vi "transmitRFID_noASK.vi"() -> ()   [LabVIEW 2015]
uses:
  <instrlib>/niUSRP/niUSRP Write Tx Data (I16).vi
panel:
  out "Loop":i32
  in  "Symbol Rate [Hz]":dbl=10000000.0 format="%#_13p"
  in  "Parameters Select":T1={"Target"=7, "Action"=0, "MemBank"=1, "truncate"=FALSE} {"MemBank" items=["00 RFU", "01 EPC", "10 TID", "11 User"]; "Action" items=["000", "001", "010", "011", "100", "101", "110", "111"]; "Target" items=["000 Inventoried (S0)", "001 Inventoried (S1)", "010 Inventoried (S2)", "011 Inventoried (S3)", "100 SL", "101 RFU", "110 RFU", "111 RFU"]}
  in  "Parameters Symbols":T2={"Tari"=2.5e-05, "PW"=0.5, "factor for \"1\" symbol"=0.5, "RTcal"=2.5, "TRcal"=2.5, "Delimiter"=1.25e-05} {"TRcal" min=1.1 max=3.0 step=0.1; "RTcal" min=2.5 max=3.0 step=0.1; "factor for \"1\" symbol" min=0.5 max=1.0 step=0.1; "PW" min=0.265 max=0.525 step=0.001; "Tari" format="%#_3p"}
  out "coerced IQ rate":dbl=100000.0 format="%#_6p"
  out "carrier frequency":dbl=100000.0 format="%#_6p"
  out "coerced gain":dbl format="%#_6f"
  out "error out":errorcluster
  in  "stop":bool
  in  "IQ rate":dbl=100000.0 format="%#_6p"
  in  "carrier frequency":dbl=100000.0 format="%#_6p"
  in  "gain":dbl format="%#_6f"
  in  "tx device names":refnum<k15>
  # "Transmit RFID"
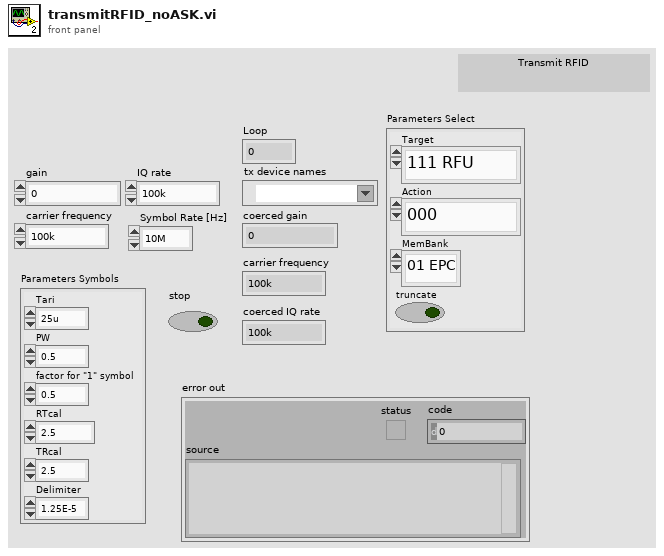
[diagram p1: front panel]
types:
  T1 = cluster{"Target":u16, "Action":u16, "MemBank":u16, "truncate":bool}
  T2 = cluster{"Tari":dbl, "PW":dbl, "factor for \"1\" symbol":dbl, "RTcal":dbl, "TRcal":dbl, "Delimiter":dbl}
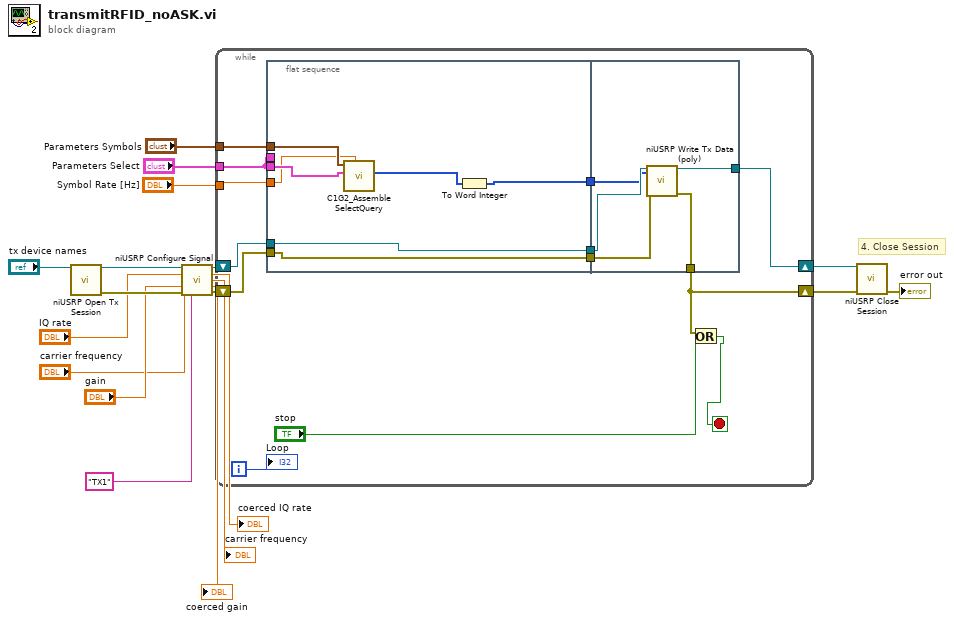
[diagram p0: block diagram]
diagram:
  # "4. Close Session"
  n1 = call <instrlib>:"niUSRP Open Tx Session.vi"("device names"="tx device names") -> ("session handle out"=w18:refnum<k15>, "error out"=w17:errorcluster)  [unwired: 13 in]
  n2 = call <instrlib>:"niUSRP Configure Signal.vi"("session handle"=w18, "IQ rate"="IQ rate", "carrier frequency"="carrier frequency", "gain"="gain", "error in (no error)"=w17, "active antenna"="TX1") -> ("session handle out"=w12:refnum<k15>, "coerced IQ rate"=→"coerced IQ rate":dbl, "coerced carrier frequency"=→"carrier frequency":dbl, "coerced gain"=→"coerced gain":dbl, "error out"=w11:errorcluster)  [unwired: 5 in]
  n3 = while {
    shift-right: [w26] -> w10
    shift-left: w12 -> [w23]
    shift-right: [w25] -> w9
    shift-left: w11 -> [w22]
    tunnel: "Parameters Symbols" -> [w27]
    tunnel: "Parameters Select" -> [w20]
    tunnel: "Symbol Rate [Hz]" -> [w28]
    i -> [w29]
    stop <- w31 stop-if-true
    n4 = flat-sequence {
      tunnel: w28 -> [w32]
      tunnel: w20 -> [w35]
      tunnel: w27 -> [w36]
      tunnel: [w38] -> w24
      tunnel: w23 -> [w38]
      tunnel: w22 -> [w37]
      tunnel: [w37] -> w21
      tunnel: w20 -> [_]
      tunnel: [w34] -> w19
      tunnel: [w43] -> w26
      tunnel: [w42] -> w25
      tunnel: w24 -> [w41]
      tunnel: w21 -> [w40]
      tunnel: w19 -> [w39]
      frame #0 {
        n5 = call "C1G2_Assemble SelectQuery.vi"("Sample Rate"=w32, "Parameters Select"=w35, "Parameters Symbols"=w36) -> ("Signal out"=w33:u8[])  [unwired: 8 in]
        n6 = To Word Integer(number=w33) -> (16bit integer=w34:i16[])
      }
      frame #1 {
        n7 = call-poly <instrlib>:"niUSRP Write Tx Data (poly).vi"("session handle"=w41, "data"=w39, "error in (no error)"=w40) -> ("session handle out"=w43:refnum<k15>, "error out"=w42:errorcluster)  [unwired: 11 in]
      }
    }
    n8 = Or(x=w25, y="stop") -> (x .or. y?=w31:bool)
    "Loop" <- w29
  }
  n9 = call <instrlib>:"niUSRP Close Session.vi"("session handle"=w10, "error in (no error)"=w9) -> ("error out"=→"error out":errorcluster)  [unwired: 13 in]
